vi "Prober_ChuckStatusCheck.vi"(8 "error in (no error)":errorcluster, 11 "ProbeStationControl in":refnum<class "ProbeStationControl.lvclass">) -> (0 "error out":errorcluster, 2 "Chuck at CONTACT?":bool=TRUE, 3 "ProbeStationControl out":refnum<class "ProbeStationControl.lvclass">)   [LabVIEW 2019, in "ProbeStationControl.lvclass"]
uses:
  ProbeStationControl.lvclass
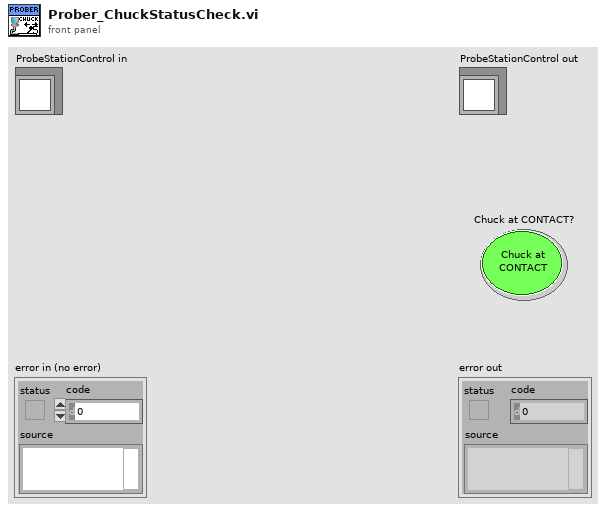
[diagram p1: front panel]
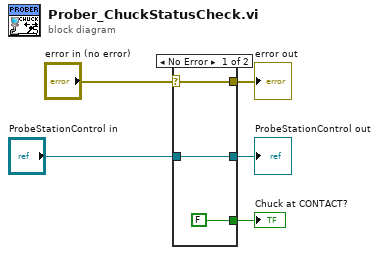
[diagram p0: block diagram]
diagram:
  n1 = case shown="No Error" "error in (no error)" {
    selector: "error in (no error)" -> [w8 w10]
    tunnel: [w8 w10] -> w4
    tunnel: "ProbeStationControl in" -> [w7 w9]
    tunnel: [FALSE _] -> w2
    tunnel: [w7 w9] -> w1
    frame No Error {
    }
    frame Error {
    }
  }
  "error out" <- w4
  "Chuck at CONTACT?" <- w2
  "ProbeStationControl out" <- w1
